vi "StringS_request.vi"(8 "error in (no error)":errorcluster, 10 "SQL request":string, 11 "DB in":refnum<class "DB.lvclass">) -> (0 "error out":errorcluster, 1 "Column Names":string[](array[string]), 2 "Result Set":string[][](table) caption="Result Set (from first statement with results)", 3 "DB out":refnum<class "DB.lvclass">)   [LabVIEW 2019, in "DB.lvclass"]
uses:
  DB.lvclass
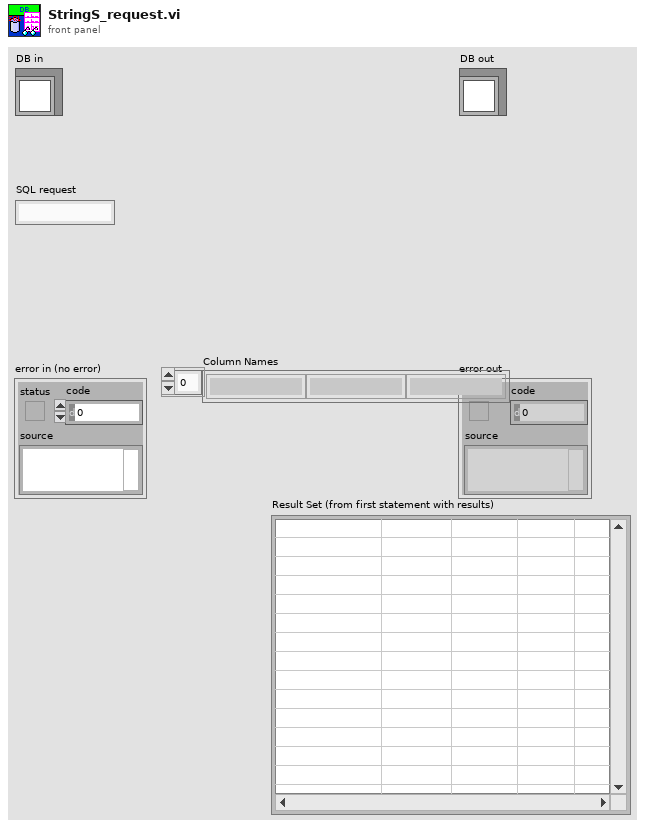
[diagram p1: front panel]
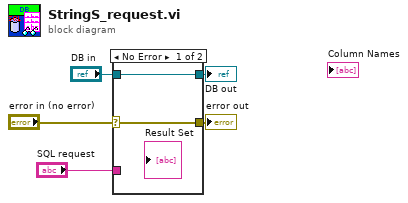
[diagram p0: block diagram]
diagram:
  n1 = case shown="No Error" "error in (no error)" {
    selector: "error in (no error)" -> [w6 w9]
    tunnel: [w6 w9] -> w4
    tunnel: [w7 w8] -> w2
    tunnel: "DB in" -> [w7 w8]
    tunnel: "SQL request" -> [_ _]
    frame No Error {
    }
    frame Error {
    }
  }
  "error out" <- w4
  "DB out" <- w2
